vi "Float64.vi"() -> ()   [LabVIEW 2015]
uses:
  <userlib>/ROS for LabVIEW Software/ROS/Code/Console/Servers/ServerSubs/TopicDef.ctl
  <userlib>/ROS for LabVIEW Software/ROS/Code/SubVIs/_ROSDirection.ctl
panel:
  out "Reply":string
  out "error out":errorcluster
  in  "Definitions":T1={"Topic"="/nums", "Type"="std_msgs/Float64", "Action"=enum."Subscriber", "Update (ms)"=1, "queue size"=1}
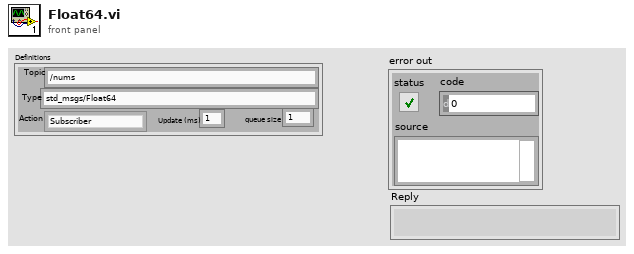
[diagram p1: front panel]
types:
  T1 = typedef "TopicDef.ctl" = cluster{"Topic":string, "Type":string, "Action":T2, "Update (ms)":u16, "queue size":u16}
  T2 = typedef "_ROSDirection.ctl" = enum16{"Node", "Publisher", "Subscriber", "ServiceClient", "ServiceProvider"}
  T3 = typedef "_ROSControl.ctl" = cluster{"topic port":u16, "Node":string, "topic":string, "type":string, "node port":u16, "error ":errorcluster, "Direction":T2, "Update (ms)":u16, "FIFO size":u16}
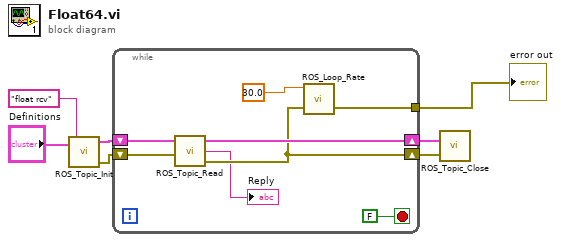
[diagram p0: block diagram]
diagram:
  n1 = call <userlib>:"ROS_Topic_Init.vi"("Definitions"="Definitions", "node"="float rcv") -> ("ROS out"=w5:T3, "error out"=w4:errorcluster)  [unwired: 1 in]
  n2 = while {
    shift-right: [w12] -> w3
    shift-left: w5 -> [w15]
    shift-right: [w11] -> w2
    shift-left: w4 -> [w14]
    tunnel: [w9] -> w1
    stop <- FALSE stop-if-true
    n3 = call <userlib>:"ROS_Topic_Read.vi"("error in (no error)"=w14, "ROS in"=w15) -> ("error out"=w11:errorcluster, "Reply"=→"Reply":string, "ROS out"=w12:T3)  [unwired: 1 in]
    n4 = call <userlib>:"ROS_Loop_Rate.vi"("Loop Rate (Hz)"=30.0, "error in"=w11) -> ("error out"=w9:errorcluster)  [unwired: 3 in, 1 out]
  }
  "error out" <- w1
  n5 = call <userlib>:"ROS_Topic_Close.vi"("error in"=w2, "ROS in"=w3) -> ()  [unwired: 2 in, 1 out]
